vi "ParseSWI.vi"(8 "error in (no error)":errorcluster, 9 "Master Device in":refnum<class "Master Device.lvclass">, 10 "Current Variables":T1[](array[typedef]), 11 "LTA-HS in":refnum<class "LTA-HS.lvclass">) -> (0 "error out":errorcluster, 2 "Master Device out":refnum<class "Master Device.lvclass">, 3 "LTA-HS out":refnum<class "LTA-HS.lvclass">)   [LabVIEW 2013, in "LTA-HS.lvclass"]
doc: "All specific devices will override ParseSWI method (i.e. you can delete the parent call)\n (1) Get devices data from private data\n (2) Get Slave Info (Ramp List) from Master Device\n (3) Parse data into \"prepared HWI\" which is in reverse order to match Ramp List."
uses:
  LTA-HS.lvclass
  TypeDefs/Active procedure variables.ctl
  Master Device/Master Device.lvclass
  ColumnVIs/SingleValMenuCol/SingleValMenuCol.lvclass
  LTA-HS.lvclass/LTA-HS.ctl
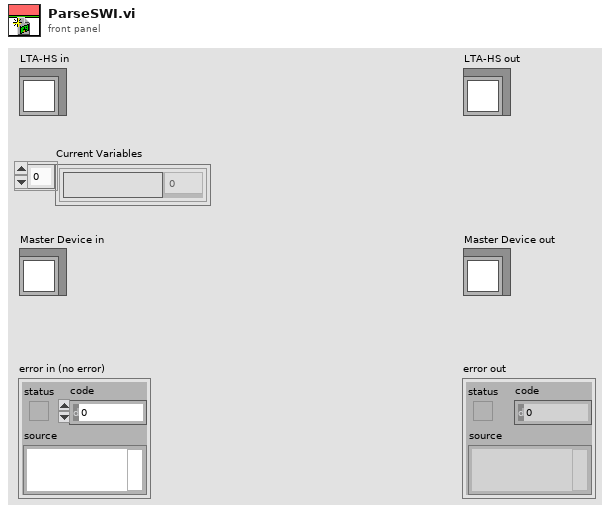
[diagram p1: front panel]
types:
  T1 = typedef "Active procedure variables.ctl" = cluster{"Procedure variable":string, "Value":dbl}
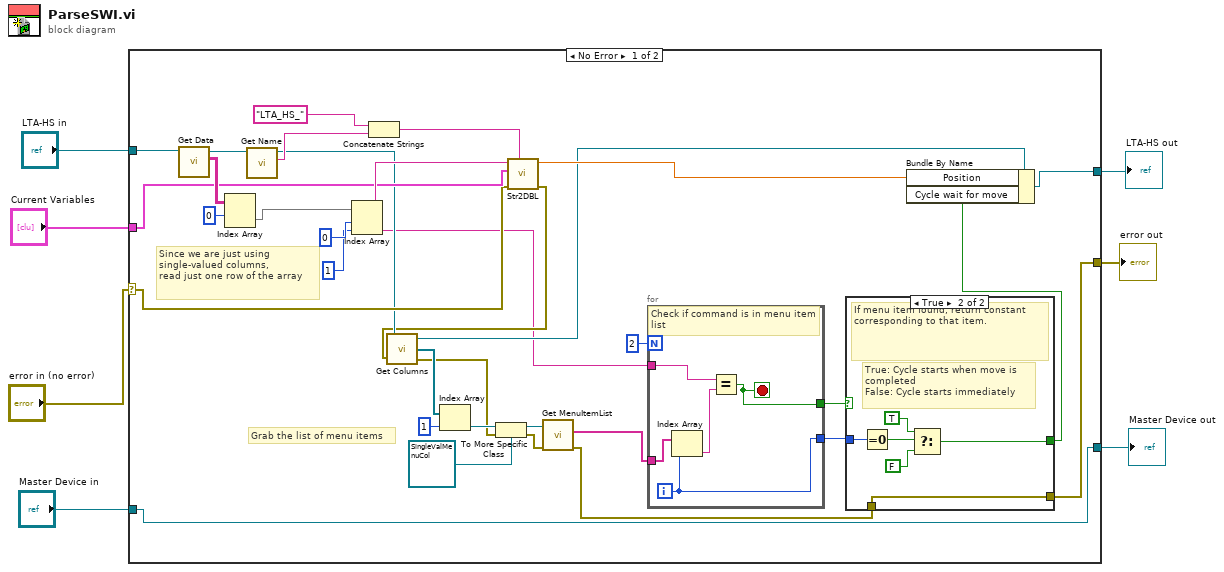
[diagram p0: block diagram]
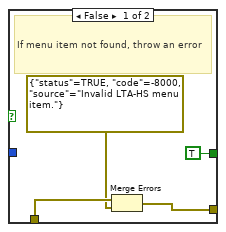
[diagram p2: hidden frame]
diagram:
  n1 = case shown="No Error" "error in (no error)" {
    selector: "error in (no error)" -> [w30 w58]
    tunnel: "LTA-HS in" -> [w41 w59]
    tunnel: "Current Variables" -> [w31 _]
    tunnel: [w28 w59] -> w4
    tunnel: [w8 w58] -> w3
    tunnel: [w27 w57] -> w2
    tunnel: "Master Device in" -> [w27 w57]
    frame No Error {
      # "Grab the list of menu items"
      # "Since we are just using single-valued columns, \nread just one row of the array"
      n2 = call-dynamic "Get Data.vi"("Device in"=w41) -> ("Table Indicator"=w40:string[][], "Device out"=w39:refnum<class "LTA-HS.lvclass">)  [unwired: 7 in, 1 out]
      n3 = Index Array(array=w40, index (row)=0) -> (element=w34:string[])  [unwired: 1 in]
      n4 = call-dynamic "Get Name.vi"("Device in"=w39) -> ("Name"=w36:string, "Device out"=w18:refnum<class "LTA-HS.lvclass">)  [unwired: 8 in, 1 out]
      n5 = Index Array(array=w34, index #1=0 ("index"), index #2=1 ("index")) -> (element #1=w32:string, element #2=w13:string)
      n6 = Concatenate Strings("LTA_HS_", w36) -> (w35:string)
      n7 = call "Str2DBL.vi"("Error Locator"=w35, "error in (no error)"=w30, "Current Variable settings"=w31, "formula"=w32) -> ("error out"=w17:errorcluster, "y value"=w29:dbl)  [unwired: 4 in]
      n8 = call-dynamic "Get Columns.vi"("Device in"=w18, "error in (no error)"=w17) -> ("Device out"=w16:refnum<class "LTA-HS.lvclass">, "Columns"=w25:refnum<class "Column.lvclass">[], "error out"=w22:errorcluster)
      n9 = Index Array(array=w25, index=1) -> (element=w23:refnum<class "Column.lvclass">)
      n10 = To More Specific Class(target class=refnum<class "SingleValMenuCol.lvclass"> refnum ("SingleValMenuCol.lvclass"), reference=w23, error in=w22) -> (specific class reference=w21:refnum<class "SingleValMenuCol.lvclass">, error out=w20:errorcluster)
      n11 = call-dynamic "Get MenuItemList.vi"("error in (no error)"=w20, "MenuCol in"=w21) -> ("error out"=w9:errorcluster, "MenuItemList"=w15:string[])  [unwired: 7 in, 1 out]
      n12 = for {
        N: 2 -> [_]
        tunnel: w15 -> [w56]
        tunnel: [w55] -> w11
        tunnel: [w53] -> w12
        tunnel: w13 -> [w52]
        i -> [w55]
        stop <- w53 stop-if-true
        # "Check if command is in menu item list"
        n13 = Index Array(array=w56, index=w55) -> (element=w54:string)
        n14 = Equal?(x=w52, y=w54) -> (x = y?=w53:bool)
      }
      n15 = case shown="True" w12 {
        tunnel: w11 -> [_ w50]
        tunnel: w9 -> [w45 w51]
        tunnel: [w43 w51] -> w8
        tunnel: [TRUE w46] -> w10
        frame False {
          # "If menu item not found, throw an error"
          n16 = Merge Errors(w45, errorcluster {"status"=TRUE, "code"=-8000, "source"="Invalid LTA-HS menu item."} ("error out")) -> (w43:errorcluster)
        }
        frame True {
          # "True: Cycle starts when move is \ncompleted \nFalse: Cycle starts immediately"
          # "If menu item found, return constant corresponding to that item."
          n17 = Equal To 0?(x=w50) -> (x = 0?=w49:bool)
          n18 = Select(t=TRUE, s=w49, f=FALSE) -> (s? t:f=w46:bool)
        }
      }
      n19 = Bundle By Name(cluster=w16, "Position"=w29, "Cycle wait for move"=w10) -> (w28:refnum<class "LTA-HS.lvclass">)
    }
    frame Error {
    }
  }
  "error out" <- w3
  "LTA-HS out" <- w4
  "Master Device out" <- w2
